vi "Joystick Control.vi"() -> ()   [LabVIEW 2014]
uses:
  <vilib>/Rock Robotics/WPI/Joystick/WPI_JoystickDeviceEnum.ctl
panel:
  out "Joystick 2":T1
  out "Joystick 1":T1
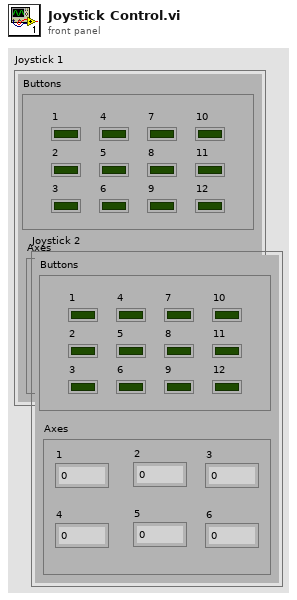
[diagram p1: front panel]
types:
  T1 = cluster{"Buttons":cluster{"1":bool, "2":bool, "3":bool, "4":bool, "5":bool, "6":bool, "7":bool, "8":bool, "9":bool, "10":bool, "11":bool, "12":bool}, "Axes":cluster{"1":dbl, "3":dbl, "2":dbl, "4":dbl, "5":dbl, "6":dbl}}
  T2 = typedef "WPI_JoystickDeviceEnum.ctl" = enum16{"USB 0", "USB 1", "USB 2", "USB 3", "USB 4", "USB 5"}
  T3 = typedef "WPI_JoystickDevRef.ctl" = cluster{"Device":T2}
  T4 = cluster{"JoystickDevRef":T3, "JoystickDevRef":T3}
  T5 = cluster{"1":bool, "2":bool, "3":bool, "4":bool, "5":bool, "6":bool, "7":bool, "8":bool, "9":bool, "10":bool, "11":bool, "12":bool}
  T6 = cluster{"1":dbl, "3":dbl, "2":dbl, "4":dbl, "5":dbl, "6":dbl}
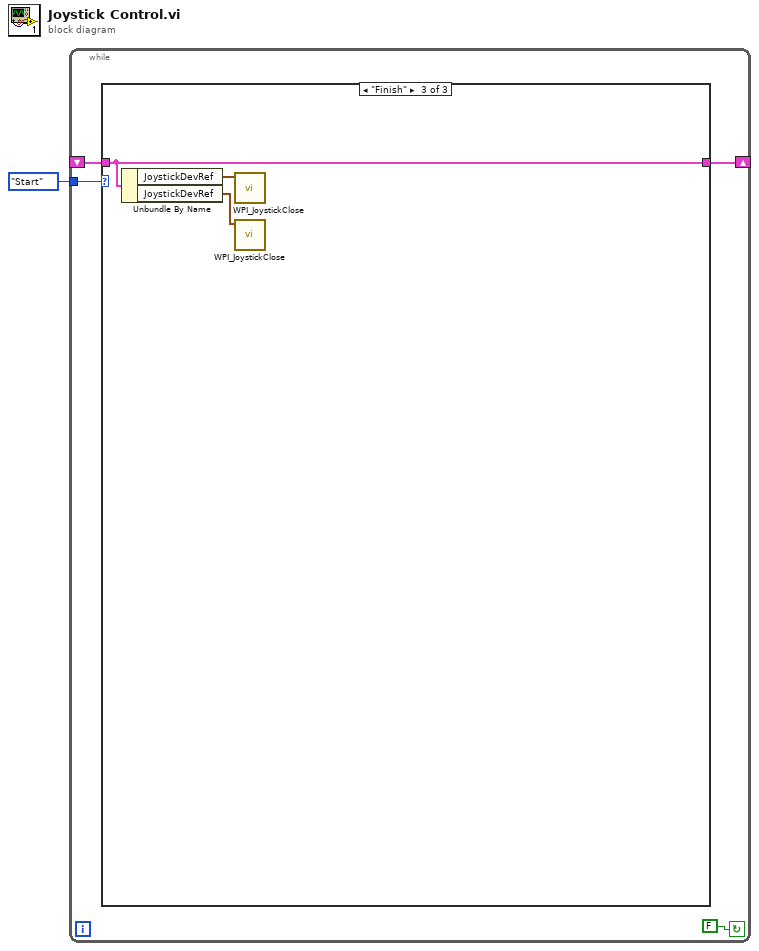
[diagram p0: block diagram]
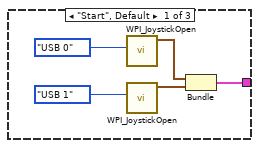
[diagram p2: hidden frame]
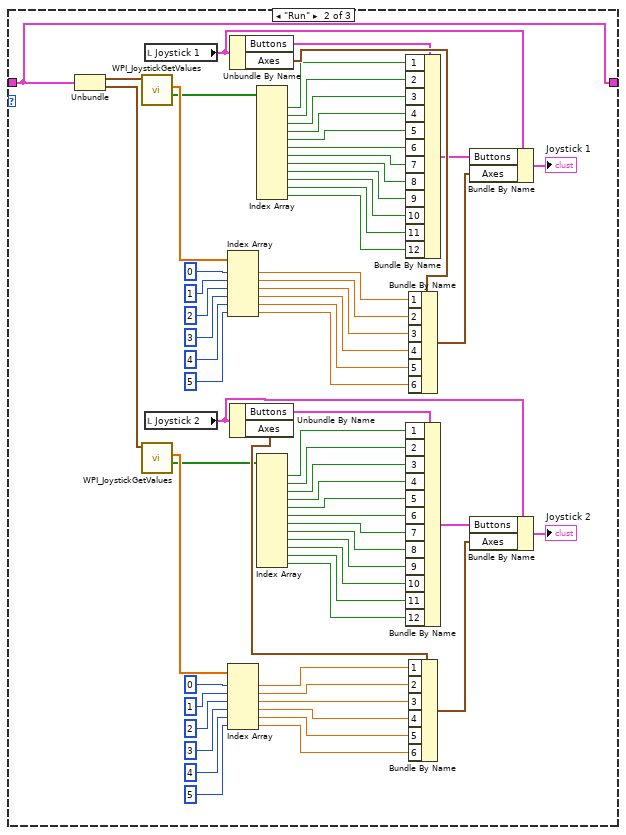
[diagram p3: hidden frame]
diagram:
  n1 = while {
    tunnel: enum8{"Start", "Run", "Finish"}."Start" ("Mode") -> [w4]
    shift-right: [w3] -> _
    shift-left: _ -> [w2]
    stop <- FALSE continue-if-true
    n2 = case shown="\"Finish\"" w4 {
      tunnel: [w6 w77 w78] -> w3
      tunnel: w2 -> [_ w77 w78]
      frame "Start", Default {
        n3 = call <vilib>:"WPI_JoystickOpen.vi"("JoystickDevice"=WPI_JoystickDeviceEnum."USB 0") -> ("JoystickDevRef"=w9:T3)  [unwired: 10 in]
        n4 = call <vilib>:"WPI_JoystickOpen.vi"("JoystickDevice"=WPI_JoystickDeviceEnum."USB 1") -> ("JoystickDevRef"=w7:T3)  [unwired: 10 in]
        n5 = Bundle("JoystickDevRef"=w9, "JoystickDevRef"=w7) -> (w6:T4)  [unwired: 1 in]
      }
      frame "Run" {
        n6 = Unbundle(w77) -> ("JoystickDevRef"=w76:T3, "JoystickDevRef"=w11:T3)
        n7 = call <vilib>:"WPI_JoystickGetValues.vi"("JoystickDevRef"=w76) -> ("Buttons"=w58:bool[], "Axes"=w72:dbl[])  [unwired: 6 in, 3 out]
        n8 = call <vilib>:"WPI_JoystickGetValues.vi"("JoystickDevRef"=w11) -> ("Buttons"=w26:bool[], "Axes"=w40:dbl[])  [unwired: 6 in, 3 out]
        n9 = local read "Joystick 1"() -> (w74:T1)
        n10 = local read "Joystick 2"() -> (w42:T1)
        n11 = Index Array(array=w72, index #1=0 ("index"), index #2=1 ("index"), index #3=2 ("index"), index #4=3 ("index"), index #5=4 ("index"), index #6=5 ("index")) -> (element #1=w65:dbl, element #2=w64:dbl, element #3=w63:dbl, element #4=w62:dbl, element #5=w61:dbl, element #6=w60:dbl)
        n12 = Index Array(array=w40, index #1=0 ("index"), index #2=1 ("index"), index #3=2 ("index"), index #4=3 ("index"), index #5=4 ("index"), index #6=5 ("index")) -> (element #1=w33:dbl, element #2=w32:dbl, element #3=w31:dbl, element #4=w30:dbl, element #5=w29:dbl, element #6=w28:dbl)
        n13 = Unbundle By Name(w74) -> ("Buttons"=w57:T5, "Axes"=w73:T6)
        n14 = Unbundle By Name(w42) -> ("Buttons"=w25:T5, "Axes"=w41:T6)
        n15 = Index Array(array=w58) -> (element #1=w56:bool, element #2=w55:bool, element #3=w54:bool, element #4=w53:bool, element #5=w52:bool, element #6=w51:bool, element #7=w50:bool, element #8=w48:bool, element #9=w49:bool, element #10=w47:bool, element #11=w46:bool, element #12=w45:bool)  [unwired: 12 in]
        n16 = Index Array(array=w26) -> (element #1=w24:bool, element #2=w23:bool, element #3=w22:bool, element #4=w21:bool, element #5=w20:bool, element #6=w19:bool, element #7=w18:bool, element #8=w16:bool, element #9=w17:bool, element #10=w15:bool, element #11=w14:bool, element #12=w13:bool)  [unwired: 12 in]
        n17 = Bundle By Name(cluster=w57, "1"=w56, "2"=w55, "3"=w54, "4"=w53, "5"=w52, "6"=w51, "7"=w50, "8"=w48, "9"=w49, "10"=w47, "11"=w46, "12"=w45) -> (w44:T5)
        n18 = Bundle By Name(cluster=w25, "1"=w24, "2"=w23, "3"=w22, "4"=w21, "5"=w20, "6"=w19, "7"=w18, "8"=w16, "9"=w17, "10"=w15, "11"=w14, "12"=w13) -> (w12:T5)
        n19 = Bundle By Name(cluster=w73, "1"=w65, "2"=w64, "3"=w63, "4"=w62, "5"=w61, "6"=w60) -> (w59:T6)
        n20 = Bundle By Name(cluster=w41, "1"=w33, "2"=w32, "3"=w31, "4"=w30, "5"=w29, "6"=w28) -> (w27:T6)
        n21 = Bundle By Name(cluster=w74, "Buttons"=w44, "Axes"=w59) -> (→"Joystick 1":T1)
        n22 = Bundle By Name(cluster=w42, "Buttons"=w12, "Axes"=w27) -> (→"Joystick 2":T1)
      }
      frame "Finish" {
        n23 = Unbundle By Name(w78) -> ("JoystickDevRef"=w80:T3, "JoystickDevRef"=w79:T3)
        n24 = call <vilib>:"WPI_JoystickClose.vi"("JoystickDevRef"=w80) -> ()  [unwired: 11 in]
        n25 = call <vilib>:"WPI_JoystickClose.vi"("JoystickDevRef"=w79) -> ()  [unwired: 11 in]
      }
    }
  }
